vi "LSCI_7-2.vi"() -> ()   [LabVIEW 2019]
uses:
  Control 2.ctl
  Settings.ctl
  <vilib>/DAQmx/write.llb/DAQmx Write (Analog DBL 1Chan 1Samp).vi
  <vilib>/DAQmx/write.llb/DAQmx Write (Analog Wfm 1Chan NSamp).vi
  <vilib>/DAQmx/write.llb/DAQmx Write (Digital 1D U32 1Chan NSamp).vi
  <vilib>/DAQmx/read.llb/DAQmx Read (Counter DBL 1Chan 1Samp).vi
  <vilib>/DAQmx/create/channels.llb/DAQmx Create Channel (AO-Voltage-Basic).vi
  <vilib>/DAQmx/create/channels.llb/DAQmx Create Channel (CI-Count Edges).vi
  <vilib>/DAQmx/miscellaneous.llb/DAQmx Fill In Error Info.vi
  <vilib>/DAQmx/create/channels.llb/DAQmx Create Channel (DO-Digital Output).vi
  <vilib>/DAQmx/configure/timing.llb/DAQmx Timing (Sample Clock).vi
  <resource>/objmgr/daqmx.rc
panel:
  in  "base path":path
  in  "Delay end (ms)":dbl=54.5
  out "Stimulation":bool=TRUE
  out "Running":bool=TRUE
  in  "STOP":bool
  out "path":path=path "D:/Haad/Whisker-tracking/v007.avi"
  in  "Whisker Cam Path":path=path "D:/Haad/Whisker-tracking/v00"
  in  "Color vs Monochrome":string="Y800 (720x540)"
  in  "ICImagingControl":refnum<k7>(container)
  in  "AOM Voltage":dbl=0.12 format="%0.3f"
  out "String 7":string="AOM Settings"
  out "String 6":string="Stroke Settings"
  out "String 5":string="Intrinsic Imaging"
  in  "LED 625 nm":bool
  in  "LED 580 nm":bool
  out "Trial #":i32=7
  out "Frames acquired":dbl=809.0 format="%0.2f"
  out "Number of Samples (Total)":dbl=10000.0
  out "Period (ms)":dbl=6.5
  out "String 4":string="Experimental Summary"
  out "String 3":string="Stimulation Control"
  out "String 2":string="Sequence Control"
  out "String":string="Trials Control"
  in  "Strength (V)":dbl=9.0
  in  "# of stimulations":i32=2
  in  "Delay (ms)":dbl=35.0
  in  "Width of pulse (ms)":dbl=80.0
  in  "# of Sequences":dbl=120.0
  in  "Sampling Rate (Hz)":T1=100000.0 format="%#_9f"
  in  "Frames/Seq":i32=7
  in  "Exposure Width (ms)":T1=5.0 format="%#_9f"
  in  "Time Between (ms)":T2=1.5 format="%#_9f"
  in  "Pre-stimulus Time":dbl=2.0 format="%.6f"
  in  "Time b/w Trials (s)":dbl=10.0 caption="Delay Time (s)"
  in  "# Trials":i32=100
  in  "Time domain signal":enum32{"Trigger Sequence", "Stimulation pulse"}(tab)
  out "LSCI Sequence":cluster{i32, dbl, dbl[]}(graph)={0, 1e-05, array[10000 elements]}
  out "Whisker Stimulus Pulse":cluster{dbl[], dbl[]}(graph)
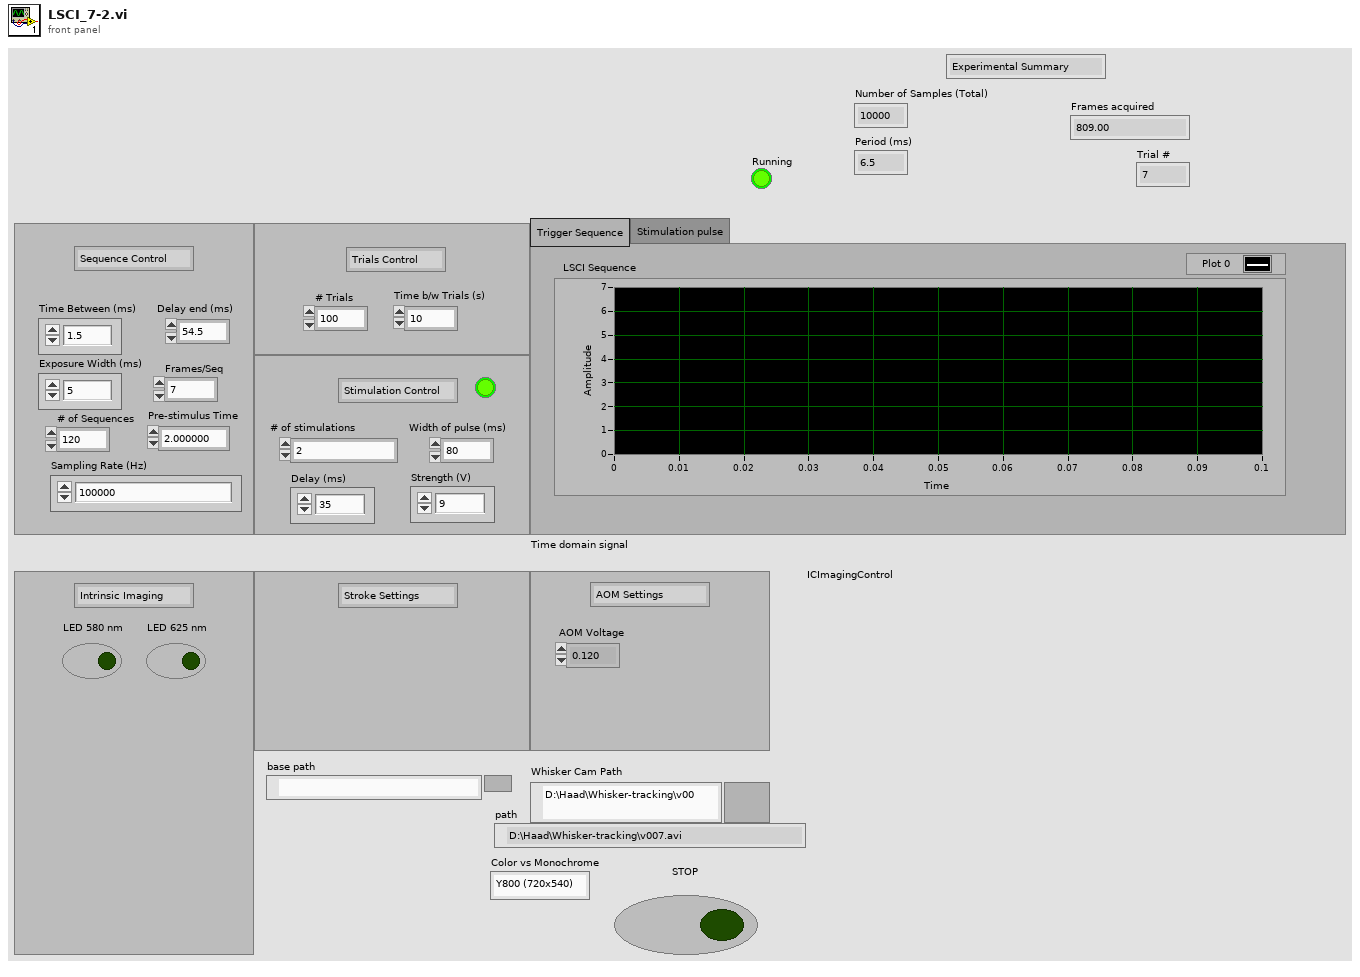
[diagram p1: front panel]
types:
  T1 = typedef "Settings.ctl" = dbl
  T2 = typedef "Control 2.ctl" = dbl
  T3 = typedef "IMAQ AVI2 Refnum.ctl" = refnum<k20>
  T4 = typedef "IMAQ Image.ctl" = refnum<image>
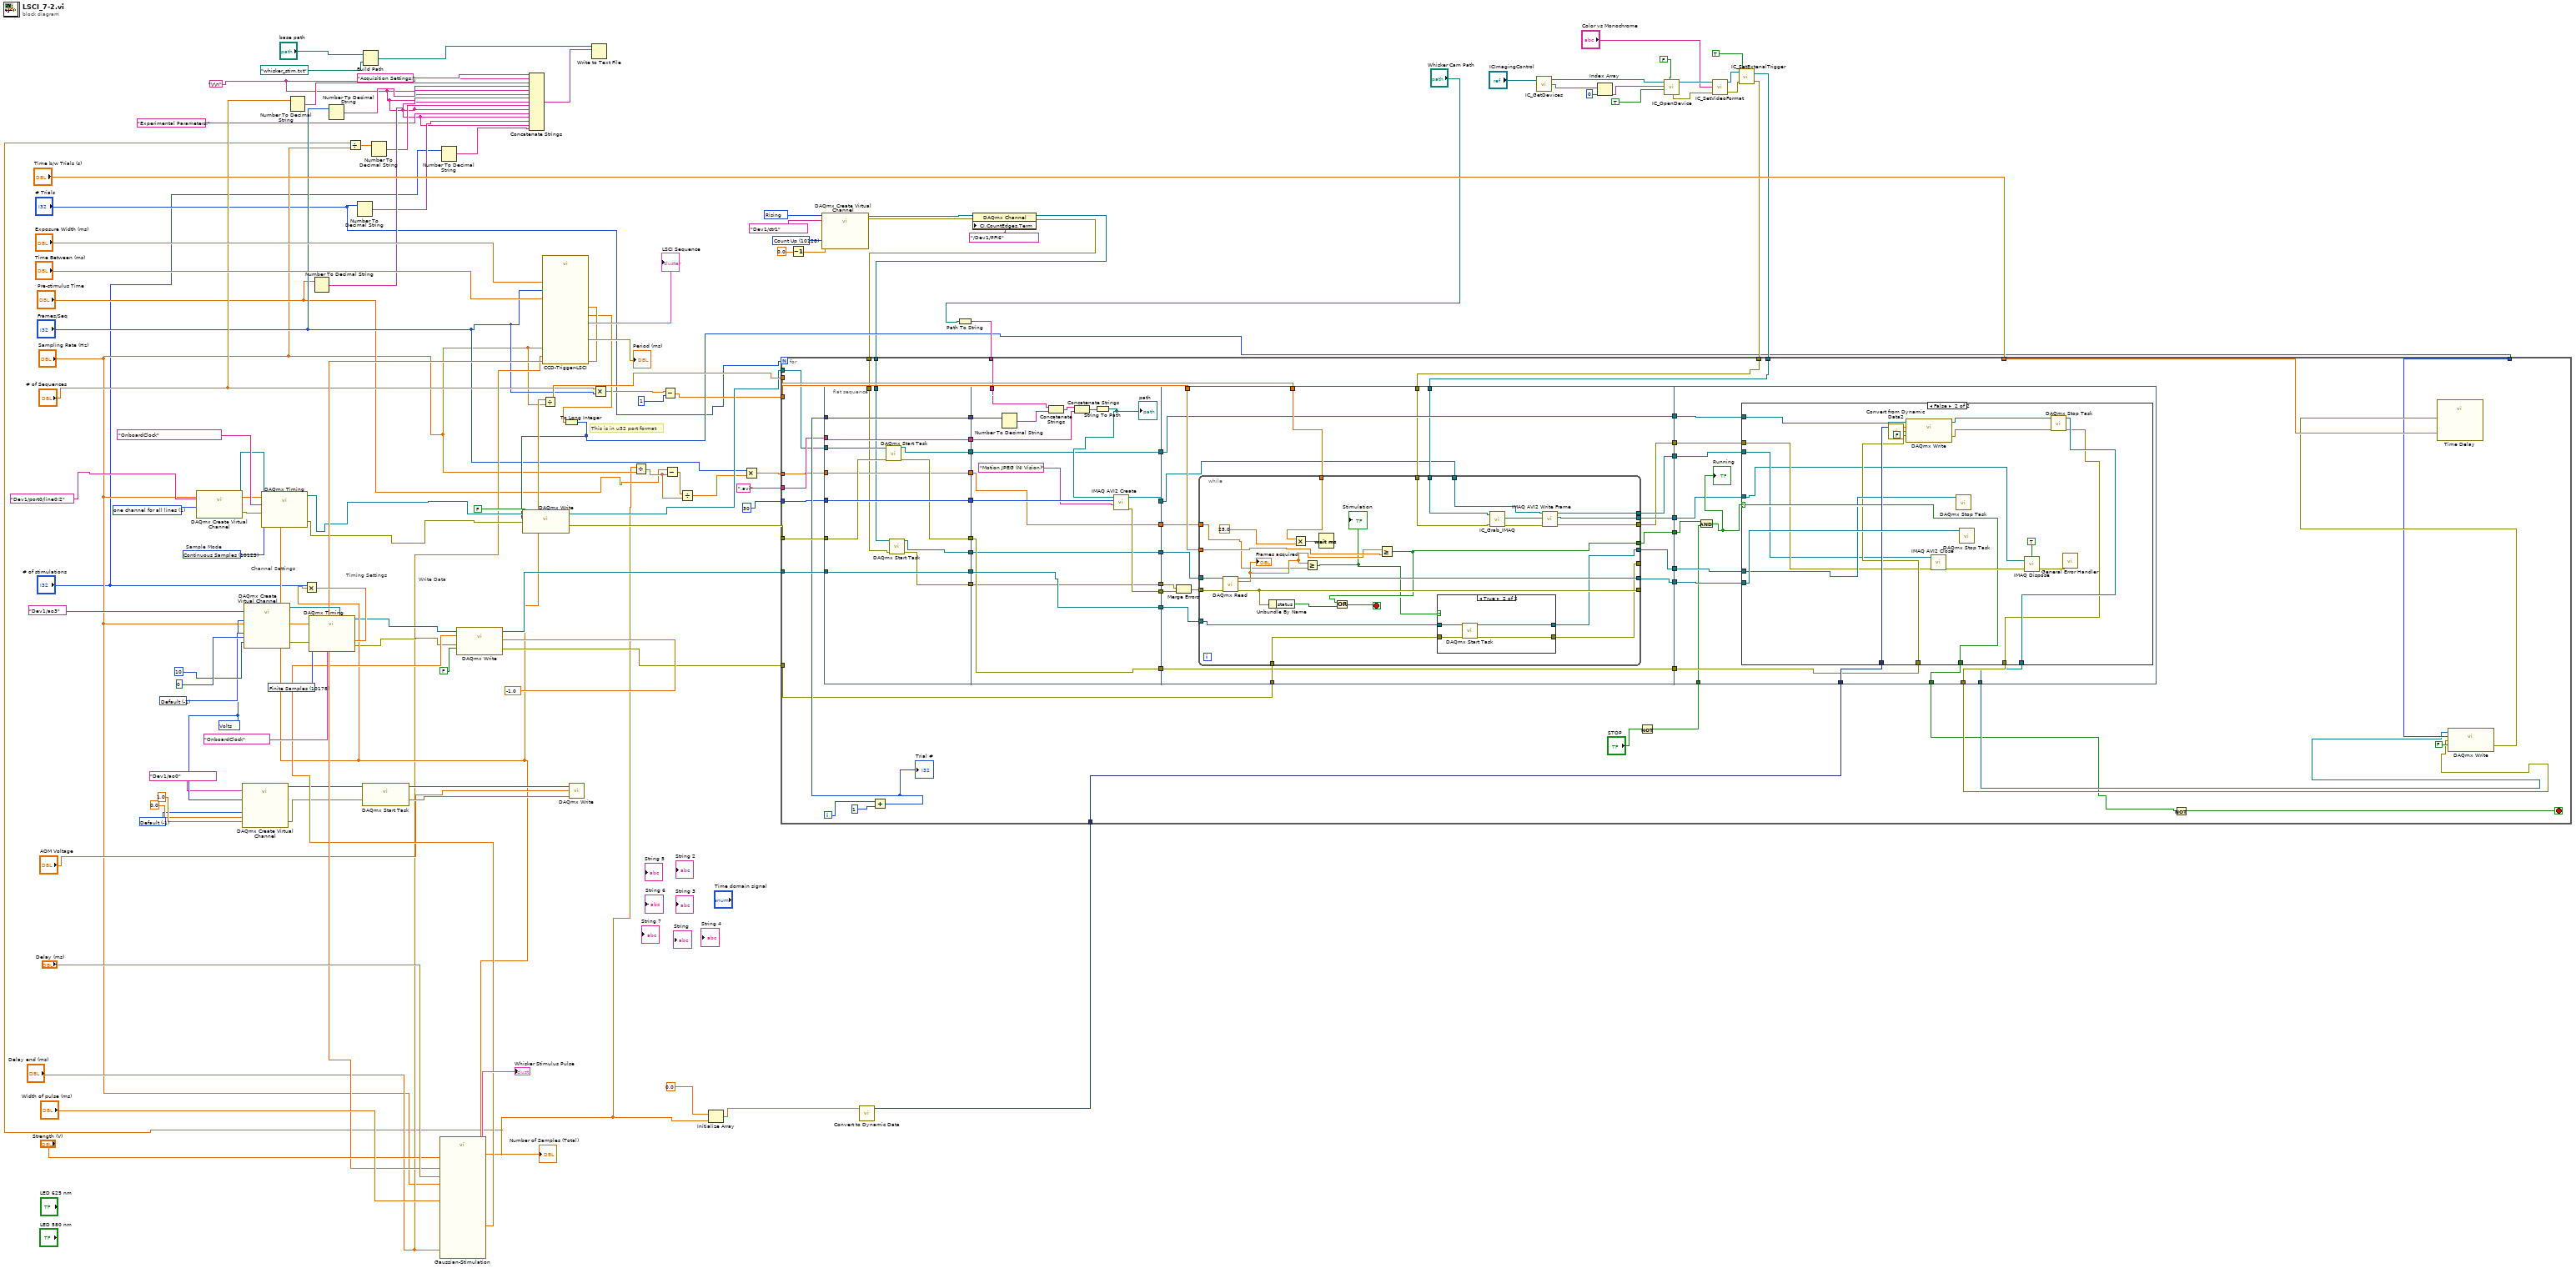
[diagram p0: block diagram]
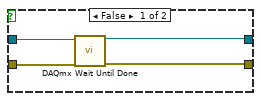
[diagram p2: hidden frame]
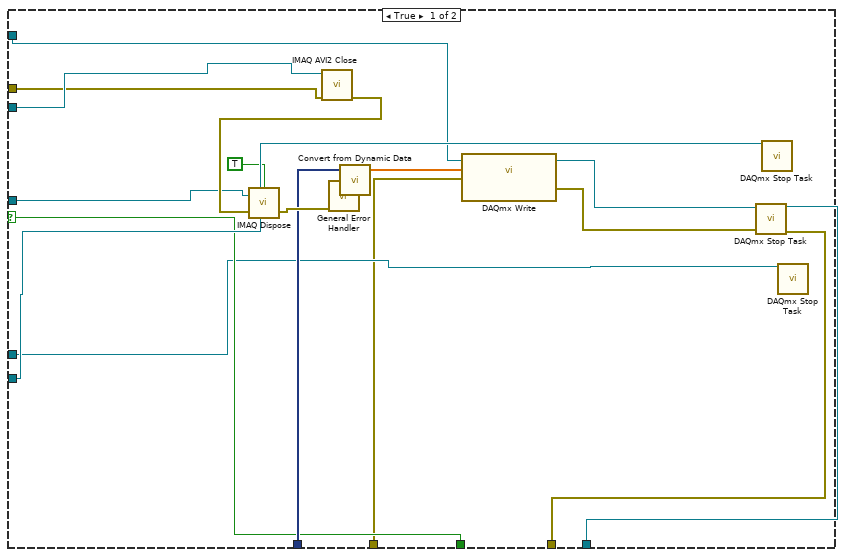
[diagram p3: hidden frame]
diagram:
  w4 = "\r\n"
  w34 = 1 items=["one channel for each line", "one channel for all lines"] ("line grouping")
  w71 = -1 items=["Default"=-1, "RSE"=10083, "Differential"=10106, "Pseudodifferential"=12529] ("output terminal configuration")
  w82 = 10280 items=["Rising"=10280, "Falling"=10171] ("edge")
  w86 = 10128 items=["Count Up"=10128, "Count Down"=10124, "Externally Controlled"=10326] ("count direction")
  w106 = 10178 items=["Finite Samples"=10178, "Continuous Samples"=10123] ("sample mode")
  w107 = -1 items=["Default"=-1, "RSE"=10083, "Differential"=10106, "Pseudodifferential"=12529] ("output terminal configuration")
  w73 = 10348 items=["Volts"=10348, "From Custom Scale"=10065] ("units")
  w112 = 10123 items=["Finite Samples"=10178, "Continuous Samples"=10123, "Hardware Timed Single Point"=12522]  # Sample Mode
  # "This is in u32 port format"
  # "Timing Settings"
  # "Write Data"
  # "Channel Settings"
  n1 = call-poly <vilib>:"DAQmx Create Virtual Channel.vi"("lines"=tag "Dev1/port0/line0:2", "line grouping"=w34) -> ("task out"=w60:refnum<k21>, "error out"=w96:errorcluster)  [unwired: 12 in]
  n2 = call-poly <vilib>:"DAQmx Create Virtual Channel.vi"("maximum value"=1.0, "minimum value"=0.0, "output terminal configuration"=w71, "physical channels"=tag "Dev1/ao0", "units"=w73) -> ("task out"=w67:refnum<k21>, "error out"=w66:errorcluster)  [unwired: 9 in]
  n3 = call-poly <vilib>:"DAQmx Create Virtual Channel.vi"("maximum value"=10, "minimum value"=0, "output terminal configuration"=w107, "physical channels"=tag "Dev1/ao3", "units"=w73) -> ("task out"=w104:refnum<k21>, "error out"=w105:errorcluster)  [unwired: 9 in]
  n4 = Number To Decimal String(number="# of Sequences") -> (decimal integer string=w16:string)  [unwired: 1 in]
  n5 = Number To Decimal String(number="Pre-stimulus Time") -> (decimal integer string=w12:string)  [unwired: 1 in]
  n6 = Number To Decimal String(number="Frames/Seq") -> (decimal integer string=w14:string)  [unwired: 1 in]
  n7 = Number To Decimal String(number="# Trials") -> (decimal integer string=w5:string)  [unwired: 1 in]
  n8 = call <vilib>:"DAQmx Start Task.vi"("task/channels in"=w67, "error in"=w66) -> ("task out"=w65:refnum<k21>, "error out"=w64:errorcluster)  [unwired: 12 in]
  n9 = Build Path(base path="base path", name or relative path=path "whisker_stim.txt" ("default name")) -> (appended path=w19:path)
  n10 = Number To Decimal String(number="# of stimulations") -> (decimal integer string=w2:string)  [unwired: 1 in]
  n11 = call "CCD-Trigger-LSCI.vi"("Delay End (ms)"="Delay end (ms)", "Sampling Rate"="Sampling Rate (Hz)", "Time Between (ms)"="Time Between (ms)", "Exposure Width (ms) in"="Exposure Width (ms)", "Frames/Seq"="Frames/Seq") -> ("# Samples"=w91:T1, "Period (ms)"=→"Period (ms)":dbl, "Array out"=w33:dbl[], "LSCI Sequence"=→"LSCI Sequence":cluster{i32, dbl, dbl[]})  [unwired: 2 in, 1 out]
  n12 = call "Gaussian-Stimulation.vi"("Strength (V)"="Strength (V)", "Delay (ms)"="Delay (ms)", "# Samples in"=w91, "Delay end (ms)"="Delay end (ms)", "Width of pulse (ms)"="Width of pulse (ms)", "Sampling Rate"="Sampling Rate (Hz)") -> ("Number of Samples (Total)"=w10:dbl, "Array 2"=w90:T1[], "# Samples out"=w61:T1, "Whisker Stimulus Pulse"=→"Whisker Stimulus Pulse":cluster{dbl[], dbl[]})  [unwired: 1 in, 1 out]
  "Number of Samples (Total)" <- w10
  n13 = call-poly <vilib>:"DAQmx Timing.vi"("task/channels in"=w60, "sample mode"=w112, "samples per channel"=w61, "rate"="Sampling Rate (Hz)", "source"=tag "OnboardClock", "error in"=w96) -> ("task out"=w38:refnum<k21>, "error out"=w37:errorcluster)  [unwired: 8 in]
  n14 = Multiply(x="# of stimulations", y=w61) -> (x*y=w101:T1)
  n15 = call-poly <vilib>:"DAQmx Timing.vi"("task/channels in"=w104, "sample mode"=w106, "samples per channel"=w101, "rate"="Sampling Rate (Hz)", "source"=tag "OnboardClock", "error in"=w105) -> ("task out"=w40:refnum<k21>, "error out"=w39:errorcluster)  [unwired: 1 in, 7 out]
  n16 = Divide(x=w10, y="Sampling Rate (Hz)") -> (x/y=w9:T1)
  n17 = Number To Decimal String(number=w9) -> (decimal integer string=w8:string)  [unwired: 1 in]
  n18 = call-poly <vilib>:"DAQmx Write.vi"("task/channels in"=w40, "auto start"=FALSE, "data"=w90, "timeout"=-1.0 ("Wirite Timeout"), "error in"=w39) -> ("task out"=w62:refnum<k21>, "error out"=w78:errorcluster)  [unwired: 9 out]
  n19 = Concatenate Strings("Acquisition Settings:" ("string"), w4, w16, w4, w14, w4, w12, w4, w8, w4, "Experimental Parameters:" ("string"), w4, w5, w4, w2) -> (w1:string)
  n20 = Divide(x=w61, y="Sampling Rate (Hz)") -> (x/y=w77:T1)
  n21 = To Long Integer(number=w33) -> (32bit integer=w32:i32[])
  n22 = call-poly <vilib>:"DAQmx Write.vi"("task/channels in"=w38, "auto start"=FALSE, "data"=w32, "error in"=w37) -> ("task out"=w36:refnum<k21>, "error out"=w79:errorcluster)  [unwired: 9 in, 1 out]
  n23 = call-poly <vilib>:"DAQmx Write.vi"("task/channels in"=w65, "data"="AOM Voltage", "error in"=w64) -> ()  [unwired: 10 in, 3 out]
  n24 = Write to Text File(file (use dialog)=w19, text=w1) -> ()  [unwired: 2 in, 3 out]
  n25 = Multiply(x="# of Sequences", y="Frames/Seq") -> (x*y=w26:dbl)
  n26 = Divide(x=w10, y="Sampling Rate (Hz)") -> (x/y=w30:T1)
  n27 = Subtract(x=w26, y=1) -> (x-y=w24:dbl)
  n28 = Subtract(x="Pre-stimulus Time", y=w30) -> (x-y=w31:T1)
  n29 = Divide(x=w31, y=w30) -> (x/y=w29:T1)
  n30 = Initialize Array(0.0 ("element"), w10) -> (w69:dbl[])
  n31 = Multiply(x="Frames/Seq", y=w29) -> (x*y=w35:T1)
  n32 = Decrement(x=0.0) -> (x-1=w85:dbl)
  n33 = call-poly <vilib>:"DAQmx Create Virtual Channel.vi"("initial count"=w85, "count direction"=w86, "edge"=w82, "counter"=tag "Dev1/ctr1") -> ("task out"=w83:refnum<k21>, "error out"=w84:errorcluster)  [unwired: 10 in]
  n34 = call "Convert to Dynamic Data"("Array"=w69) -> ("Dynamic Data Type"=w68:dynamicdata)  [unwired: 3 in]
  n35 = Path To String(path="Whisker Cam Path") -> (string=w44:string)
  n36 = property class="DAQmx Channel"(reference=w83, error in=w84, "CI.CountEdges.Term"=tag "/Dev1/PFI6") -> (reference out=w27:refnum<k21>, error out=w28:errorcluster)
  n37 = call <userlib>:"IC_GetDevices.vi"("ICImagingControl In"="ICImagingControl") -> ("ICImagingControl Out"=w56:refnum<k7>, "Devices"=w55:string[])  [unwired: 1 in, 1 out]
  n38 = Index Array(array=w55, index=0) -> (element=w53:string)
  n39 = call <userlib>:"IC_OpenDevice.vi"("Color"=FALSE, "Live"=TRUE, "Device"=w53, "ICImagingControl In"=w56) -> ("ICImagingControl Out"=w52:refnum<k7>, "Error Out"=w50:errorcluster)  [unwired: 2 in, 4 out]
  n40 = call <userlib>:"IC_SetVideoFormat.vi"("Error In (no error)"=w50, "VideoFormat"="Color vs Monochrome", "ICImagingControl In"=w52) -> ("Error Out"=w48:errorcluster, "ICImagingControl Out"=w49:refnum<k7>)  [unwired: 1 out]
  n41 = call <userlib>:"IC_SetExtenalTrigger.vi"("Error In (no error)"=w48, "Trigger"=TRUE, "ICImagingControl In"=w49) -> ("Error Out"=w47:errorcluster, "ICImagingControl Out"=w46:refnum<k7>)
  n42 = for {
    N: "# Trials" -> [_]
    tunnel: w79 -> [w165]
    tunnel: w62 -> [w164]
    tunnel: w78 -> [w137]
    tunnel: w36 -> [w141]
    tunnel: w77 -> [w163]
    tunnel: w24 -> [w162]
    tunnel: "Time b/w Trials (s)" -> [w159]
    tunnel: w68 -> [w151]
    tunnel: w32 -> [w156]
    tunnel: w47 -> [w115]
    tunnel: w46 -> [w116]
    tunnel: w44 -> [w154]
    tunnel: ".avi" ("string") -> [w153]
    tunnel: u32 30 ("Frames Per Second") -> [w152]
    tunnel: w35 -> [w133]
    tunnel: w28 -> [w125]
    tunnel: w27 -> [w124]
    i -> [w161]
    stop <- w139 stop-if-true
    n43 = flat-sequence {
      tunnel: w152 -> [w175]
      tunnel: w153 -> [w176]
      tunnel: w155 -> [w177]
      tunnel: w164 -> [w178]
      tunnel: w165 -> [w173]
      tunnel: [w172] -> w146
      tunnel: [w178] -> w145
      tunnel: [w177] -> w144
      tunnel: [w176] -> w143
      tunnel: [w175] -> w142
      tunnel: w141 -> [w174]
      tunnel: [w171] -> w140
      tunnel: [w170] -> w134
      tunnel: w133 -> [w170]
      tunnel: w125 -> [w169]
      tunnel: w124 -> [w168]
      tunnel: [w167] -> w122
      tunnel: [w166] -> w121
      tunnel: w154 -> [w193]
      tunnel: [w186] -> w132
      tunnel: w146 -> [w181]
      tunnel: w145 -> [w184]
      tunnel: w144 -> [w195]
      tunnel: w143 -> [w191]
      tunnel: w142 -> [w188]
      tunnel: w140 -> [w185]
      tunnel: [w185] -> w131
      tunnel: [w184] -> w130
      tunnel: [w183] -> w129
      tunnel: [w182] -> w128
      tunnel: w134 -> [w182]
      tunnel: [w181] -> w126
      tunnel: [w180] -> w123
      tunnel: w122 -> [w180]
      tunnel: w121 -> [w179]
      tunnel: [w179] -> w120
      tunnel: w163 -> [w215]
      tunnel: w162 -> [w214]
      tunnel: w132 -> [w198]
      tunnel: [w213] -> w150
      tunnel: [w212] -> w149
      tunnel: w131 -> [w212]
      tunnel: w137 -> [w211]
      tunnel: w130 -> [w210]
      tunnel: [w209] -> w136
      tunnel: [w208] -> w135
      tunnel: w128 -> [w207]
      tunnel: w129 -> [w206]
      tunnel: [w204] -> w127
      tunnel: w126 -> [w204]
      tunnel: w123 -> [w203]
      tunnel: w120 -> [w202]
      tunnel: [w199] -> w117
      tunnel: w116 -> [w201]
      tunnel: w115 -> [w200]
      tunnel: [w197] -> w114
      tunnel: [w196] -> w113
      tunnel: w151 -> [w263]
      tunnel: w150 -> [w262]
      tunnel: w149 -> [w261]
      tunnel: [w260] -> w148
      tunnel: [w259] -> w147
      tunnel: [w258] -> w138
      tunnel: w136 -> [w257]
      tunnel: w135 -> [w256]
      tunnel: w127 -> [w255]
      tunnel: w118 -> [w253]
      tunnel: w117 -> [w252]
      tunnel: w114 -> [w251]
      tunnel: w113 -> [w250]
      frame #0 {
        n44 = call <vilib>:"DAQmx Start Task.vi"("task/channels in"=w174, "error in"=w173) -> ("task out"=w171:refnum<k21>, "error out"=w172:errorcluster)  [unwired: 12 out]
        n45 = call <vilib>:"DAQmx Start Task.vi"("task/channels in"=w168, "error in"=w169) -> ("task out"=w167:refnum<k21>, "error out"=w166:errorcluster)  [unwired: 12 in]
      }
      frame #1 {
        n46 = Number To Decimal String(number=w195) -> (decimal integer string=w194:string)  [unwired: 1 in]
        n47 = Concatenate Strings(w193, w194) -> (w192:string)
        n48 = Concatenate Strings(w192, w191) -> (w190:string)
        n49 = String To Path(string=w190) -> (path=w189:path)
        "path" <- w189
        n50 = call "IMAQ AVI2 Create"("Codec"="Motion JPEG (NI Vision)", "Frames Per Second"=w188, "AVI Path"=w189) -> ("error out"=w183:errorcluster, "AVI Refnum"=w186:T3)  [unwired: 7 in]
      }
      frame #2 {
        n51 = Merge Errors(w202, w206) -> (w205:errorcluster)
        n52 = while {
          tunnel: w203 -> [w241]
          tunnel: w205 -> [w240]
          tunnel: [w239] -> w213
          tunnel: [w238] -> _
          tunnel: w215 -> [w237]
          tunnel: w214 -> [w230]
          tunnel: w211 -> [w233]
          tunnel: w210 -> [w234]
          tunnel: [w231] -> w209
          tunnel: [w232] -> _
          tunnel: [w226] -> w208
          tunnel: w207 -> [w225]
          tunnel: w198 -> [w221]
          tunnel: w201 -> [w220]
          tunnel: w200 -> [w219]
          tunnel: [w218] -> w199
          tunnel: [w217] -> w197
          tunnel: [w216] -> w196
          stop <- w227 stop-if-true
          n53 = call-poly <vilib>:"DAQmx Read.vi"("task/channels in"=w241, "error in"=w240) -> ("task out"=w239:refnum<k21>, "data"=w229:dbl, "error out"=w238:errorcluster)  [unwired: 11 in]
          "Frames acquired" <- w229
          n54 = Unbundle By Name(w238) -> ("status"=w228:bool)
          n55 = Multiply(x=w237, y=T1 25.0) -> (x*y=w236:T1)
          n56 = Greater Or Equal?(x=w229, y=w225) -> (x >= y?=w224:bool)
          "Stimulation" <- w224
          n57 = Wait (ms)(milliseconds to wait=w236) -> ()  [unwired: 1 out]
          n58 = Greater Or Equal?(x=w229, y=w230) -> (x >= y?=w226:bool)
          n59 = Or(x=w226, y=w228) -> (x .or. y?=w227:bool)
          n60 = case shown="True" w224 {
            tunnel: w234 -> [w245 w249]
            tunnel: w233 -> [w244 w248]
            tunnel: [w242 w247] -> w232
            tunnel: [w243 w246] -> w231
            frame False {
              n61 = call <vilib>:"DAQmx Wait Until Done.vi"("task/channels in"=w245, "error in"=w244) -> ("task out"=w243:refnum<k21>, "error out"=w242:errorcluster)  [unwired: 12 in]
            }
            frame True {
              n62 = call <vilib>:"DAQmx Start Task.vi"("task/channels in"=w249, "error in"=w248) -> ("task out"=w246:refnum<k21>, "error out"=w247:errorcluster)  [unwired: 12 out]
            }
          }
          n63 = call <userlib>:"IC_Grab_IMAQ.vi"("ICImagingControl In"=w220, "Error In (no error)"=w219) -> ("Image Out"=w223:T4, "Error Out"=w222:errorcluster)  [unwired: 1 in, 2 out]
          n64 = call "IMAQ AVI2 Write Frame"("error in (no error)"=w222, "Image"=w223, "AVI Refnum"=w221) -> ("error out"=w216:errorcluster, "Image Out (duplicate)"=w217:T4, "AVI Refnum (duplicate)"=w218:T3)  [unwired: 6 in]
        }
      }
      frame #3 {
        n65 = And(x=w256, y=w253) -> (x .and. y?=w254:bool)
        "Running" <- w254
        n66 = case shown="False" w254 {
          selector: w254 -> [w270 w287]
          tunnel: w263 -> [w275 w297]
          tunnel: w262 -> [w274 w298]
          tunnel: w261 -> [w271 w294]
          tunnel: [w273 w288] -> w260
          tunnel: [w272 w289] -> w259
          tunnel: [w270 w287] -> w258
          tunnel: w257 -> [w269 w286]
          tunnel: w255 -> [w268 w285]
          tunnel: w252 -> [w266 w282]
          tunnel: w251 -> [w265 w281]
          tunnel: w250 -> [w264 w283]
          frame True {
            n67 = call "IMAQ AVI2 Close"("error in (no error)"=w264, "AVI Refnum"=w266) -> ("error out"=w276:errorcluster)  [unwired: 9 in]
            n68 = call "IMAQ Dispose"("All Images? (No)"=TRUE, "Image"=w265, "error in (no error)"=w276) -> ("error out"=w277:errorcluster)  [unwired: 3 in]
            n69 = call <vilib>:"General Error Handler.vi"("error in (no error)"=w277) -> ()  [unwired: 10 in, 5 out]
            n70 = call "Convert from Dynamic Data"("Dynamic Data Type"=w275) -> ("Array"=w280:dbl[])  [unwired: 3 in]
            n71 = call-poly <vilib>:"DAQmx Write.vi"("task/channels in"=w271, "data"=w280, "error in"=w268) -> ("task out"=w279:refnum<k21>, "error out"=w278:errorcluster)  [unwired: 10 in, 1 out]
            n72 = call <vilib>:"DAQmx Stop Task.vi"("task/channels in"=w279, "error in"=w278) -> ("task out"=w272:refnum<k21>, "error out"=w273:errorcluster)  [unwired: 12 in]
            n73 = call <vilib>:"DAQmx Stop Task.vi"("task/channels in"=w274) -> ()  [unwired: 13 in, 2 out]
            n74 = call <vilib>:"DAQmx Stop Task.vi"("task/channels in"=w269) -> ()  [unwired: 13 in, 2 out]
          }
          frame False {
            n75 = call "Convert from Dynamic Data2"("Dynamic Data Type"=w297) -> ("Array"=w296:dbl[])  [unwired: 3 in]
            n76 = call-poly <vilib>:"DAQmx Write.vi"("task/channels in"=w294, "auto start"=FALSE, "data"=w296, "error in"=w285) -> ("task out"=w293:refnum<k21>, "error out"=w292:errorcluster)  [unwired: 9 in, 1 out]
            n77 = call "IMAQ AVI2 Close"("error in (no error)"=w283, "AVI Refnum"=w282) -> ("error out"=w291:errorcluster)  [unwired: 9 in]
            n78 = call <vilib>:"DAQmx Stop Task.vi"("task/channels in"=w286) -> ()  [unwired: 13 in, 2 out]
            n79 = call <vilib>:"DAQmx Stop Task.vi"("task/channels in"=w298) -> ()  [unwired: 13 in, 2 out]
            n80 = call "IMAQ Dispose"("All Images? (No)"=TRUE, "Image"=w281, "error in (no error)"=w291) -> ("error out"=w290:errorcluster)  [unwired: 3 in]
            n81 = call <vilib>:"DAQmx Stop Task.vi"("task/channels in"=w293, "error in"=w292) -> ("task out"=w289:refnum<k21>, "error out"=w288:errorcluster)  [unwired: 12 in]
            n82 = call <vilib>:"General Error Handler.vi"("error in (no error)"=w290) -> ()  [unwired: 10 in, 5 out]
          }
        }
      }
    }
    n83 = Add(x=w161, y=1) -> (x+y=w155:i32)
    "Trial #" <- w155
    n84 = Not(x="STOP") -> (.not. x?=w118:bool)
    n85 = Not(x=w138) -> (.not. x?=w139:bool)
    n86 = call-poly <vilib>:"DAQmx Write.vi"("task/channels in"=w147, "auto start"=FALSE, "data"=w156, "error in"=w148) -> ("error out"=w157:errorcluster)  [unwired: 9 in, 2 out]
    n87 = call "Time Delay"("error in (no error)"=w157, "Delay Time (s)"=w159) -> ()  [unwired: 9 in, 1 out]
  }
